vi "ReadAddress.vi"(0 "Task in":refnum<class "WaveformTask.lvclass">, 5 "address":u64, 11 "error in (no error)":errorcluster) -> (4 "Task out":refnum<class "WaveformTask.lvclass">, 6 "data":u64, 15 "error out":errorcluster)   [LabVIEW 2015, in "WaveformTask.lvclass"]
uses:
  WaveformTask.lvclass
  WaveformTask.lvclass/WaveformTask.ctl
  <instrlib>/_niInstr/Instruction Framework/v1/Host/Instruction Target/niInstr Instruction Target v1 Host.lvclass
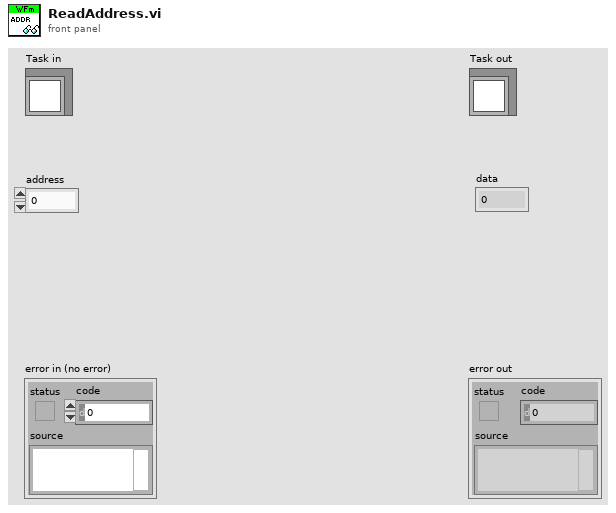
[diagram p1: front panel]
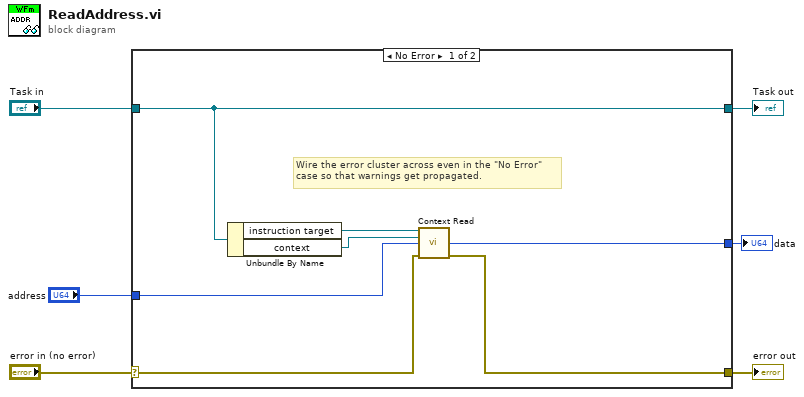
[diagram p0: block diagram]
diagram:
  n1 = case shown="No Error" "error in (no error)" {
    selector: "error in (no error)" -> [w11 w15]
    tunnel: [w10 w15] -> w5
    tunnel: [w13 w14] -> w3
    tunnel: "Task in" -> [w13 w14]
    tunnel: "address" -> [w8 _]
    tunnel: [w7 _] -> w1
    frame No Error {
      # "Wire the error cluster across even in the \"No Error\"\ncase so that warnings get propagated."
      n2 = Unbundle By Name(w13) -> ("instruction target"=w12:refnum<class "niInstr FIFO Register Bus v1 Host.lvclass">, "context"=w9:refnum<class "niInstr Instruction Framework Context v1 Host.lvclass">)
      n3 = call <instrlib>:"Context Read.vi"("instruction target in"=w12, "context in"=w9, "address"=w8, "error in"=w11) -> ("data"=w7:u64, "error out"=w10:errorcluster)  [unwired: 8 in, 2 out]
    }
    frame Error {
    }
  }
  "error out" <- w5
  "Task out" <- w3
  "data" <- w1
